vi "MultiTool-Track-Generate-ndipolarisFileOutput-Q-vectors-Accepts Joystick Command with Time Display-Testing time diff with tick.vi"() -> ()   [LabVIEW 2013]
panel:
  out "TIME":string
  out "bytes written":i32
  out "Return time string":string
  out "Length":u8
  out "Command":u8
  out "Tool 2":T1={"Port Handle"="", "Frame Number"=0, "Tx"=0.0, "Ty"=0.0, "Tz"=0.0, "Q0"=0.0, "Qx"=0.0, "Qy"=0.0, "Qz"=0.0, "Deviation"=0.0, " Markers Missing"=TRUE, "Out of Volume"=TRUE} {"Deviation" format="%#.4f"; "Qz" format="%#.4f"; "Qy" format="%#.4f"; "Qx" format="%#.4f"; "Q0" format="%#.4f"; "Tz" format="%#.2f"; "Ty" format="%#.2f"; "Tx" format="%#.2f"}
  in  "Location of ROM File for Tool 2":path=path "C:/Program Files (x86)/Northern Digital Inc/8700339.rom"
  in  "NDI  Running":bool=TRUE
  out "Stop Reading":bool=TRUE
  out "Start Reading":bool
  out "Object Identifier":string="0"
  in  "Track Outside Measurement Volume? (F:No)":bool
  in  "Track Stray Markers? (F:No)":bool
  out "Tool 1":T1={"Port Handle"="", "Frame Number"=0, "Tx"=0.0, "Ty"=0.0, "Tz"=0.0, "Q0"=0.0, "Qx"=0.0, "Qy"=0.0, "Qz"=0.0, "Deviation"=0.0, " Markers Missing"=TRUE, "Out of Volume"=TRUE} {"Deviation" format="%#.4f"; "Qz" format="%#.4f"; "Qy" format="%#.4f"; "Qx" format="%#.4f"; "Q0" format="%#.4f"; "Tz" format="%#.2f"; "Ty" format="%#.2f"; "Tx" format="%#.2f"}
  out "TCP loop":i32
  in  "TCP Server Running":bool=TRUE
  in  "Output Directory":path=path "C:/Users/Diogo/Desktop/NDI-Labview Gripper"
  out "NDI Loop":i32
  in  "VISA resource name":refnum<visa-resource-name>="COM8"
  in  "Reset? (T:Yes)":bool=TRUE
  in  "Location of ROM File for Tool 1":path=path "C:/Program Files (x86)/Northern Digital Inc/8700449.rom"
  in  "Serial Configuration":T2={"Baud Rate (9600)"=9600, "Flow Control (0:None)"=0, "Parity"=0, "Data Bits"=8, "Stop Bits"=10} {"Stop Bits" items=["1.0"=10, "2.0"=20]; "Parity" items=["None", "Odd", "Even"]; "Flow Control (0:None)" items=["None", "XON/XOFF"]; "Baud Rate (9600)" items=["9600"=9600, "14.4k"=14400, "19.2k"=19200, "38.4k"=38400, "57.6k "=57600, "115.2k"=115200]}
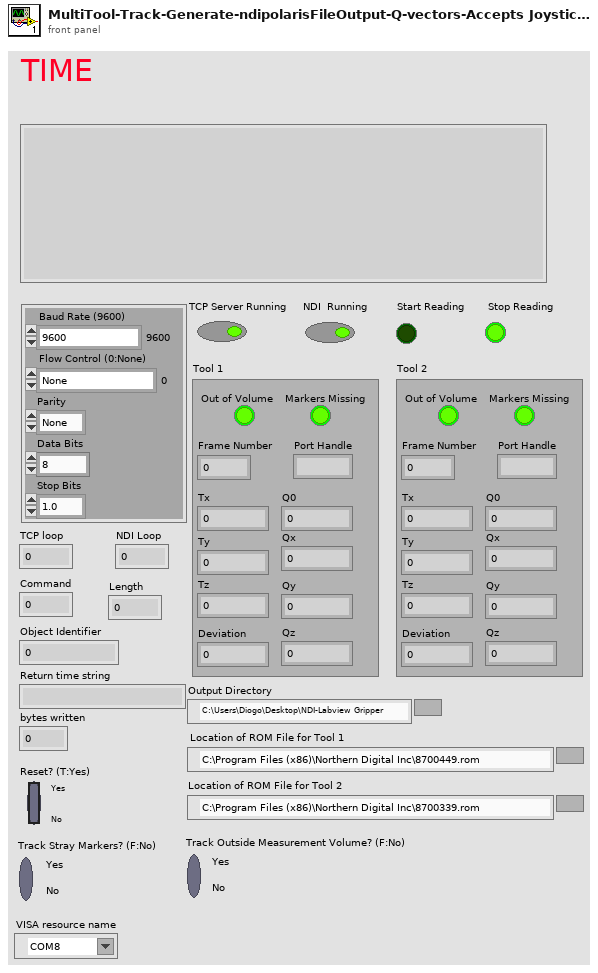
[diagram p1: front panel]
types:
  T1 = cluster{"Port Handle":string, "Frame Number":i32, "Tx":dbl, "Ty":dbl, "Tz":dbl, "Q0":dbl, "Qx":dbl, "Qy":dbl, "Qz":dbl, "Deviation":dbl, " Markers Missing":bool, "Out of Volume":bool}
  T2 = cluster{"Baud Rate (9600)":u32, "Flow Control (0:None)":u16, "Parity":u16, "Data Bits":u16, "Stop Bits":u16}
  T3 = cluster{"Port Handle":string, "Frame Number":u32, "Tx":dbl, "Ty":dbl, "Tz":dbl, "Q0":dbl, "Qx":dbl, "Qy":dbl, "Qz":dbl, "Deviation":dbl, "Missing?":bool, "Out of Volume?":bool}[]
  T4 = cluster{"Transformations[0]":cluster{"Port Handle":string, "Frame Number":u32, "Tx":dbl, "Ty":dbl, "Tz":dbl, "Q0":dbl, "Qx":dbl, "Qy":dbl, "Qz":dbl, "Deviation":dbl, "Missing?":bool, "Out of Volume?":bool}, "Transformations[1]":cluster{"Port Handle":string, "Frame Number":u32, "Tx":dbl, "Ty":dbl, "Tz":dbl, "Q0":dbl, "Qx":dbl, "Qy":dbl, "Qz":dbl, "Deviation":dbl, "Missing?":bool, "Out of Volume?":bool}, "Transformations[2]":cluster{"Port Handle":string, "Frame Number":u32, "Tx":dbl, "Ty":dbl, "Tz":dbl, "Q0":dbl, "Qx":dbl, "Qy":dbl, "Qz":dbl, "Deviation":dbl, "Missing?":bool, "Out of Volume?":bool}, "Transformations[3]":cluster{"Port Handle":string, "Frame Number":u32, "Tx":dbl, "Ty":dbl, "Tz":dbl, "Q0":dbl, "Qx":dbl, "Qy":dbl, "Qz":dbl, "Deviation":dbl, "Missing?":bool, "Out of Volume?":bool}, "Transformations[4]":cluster{"Port Handle":string, "Frame Number":u32, "Tx":dbl, "Ty":dbl, "Tz":dbl, "Q0":dbl, "Qx":dbl, "Qy":dbl, "Qz":dbl, "Deviation":dbl, "Missing?":bool, "Out of Volume?":bool}, "Transformations[5]":cluster{"Port Handle":string, "Frame Number":u32, "Tx":dbl, "Ty":dbl, "Tz":dbl, "Q0":dbl, "Qx":dbl, "Qy":dbl, "Qz":dbl, "Deviation":dbl, "Missing?":bool, "Out of Volume?":bool}, "Transformations[6]":cluster{"Port Handle":string, "Frame Number":u32, "Tx":dbl, "Ty":dbl, "Tz":dbl, "Q0":dbl, "Qx":dbl, "Qy":dbl, "Qz":dbl, "Deviation":dbl, "Missing?":bool, "Out of Volume?":bool}, "Transformations[7]":cluster{"Port Handle":string, "Frame Number":u32, "Tx":dbl, "Ty":dbl, "Tz":dbl, "Q0":dbl, "Qx":dbl, "Qy":dbl, "Qz":dbl, "Deviation":dbl, "Missing?":bool, "Out of Volume?":bool}, "Transformations[8]":cluster{"Port Handle":string, "Frame Number":u32, "Tx":dbl, "Ty":dbl, "Tz":dbl, "Q0":dbl, "Qx":dbl, "Qy":dbl, "Qz":dbl, "Deviation":dbl, "Missing?":bool, "Out of Volume?":bool}}
  T5 = cluster{"Port Handle":string, "Frame Number":u32, "Tx":dbl, "Ty":dbl, "Tz":dbl, "Q0":dbl, "Qx":dbl, "Qy":dbl, "Qz":dbl, "Deviation":dbl, "Missing?":bool, "Out of Volume?":bool}
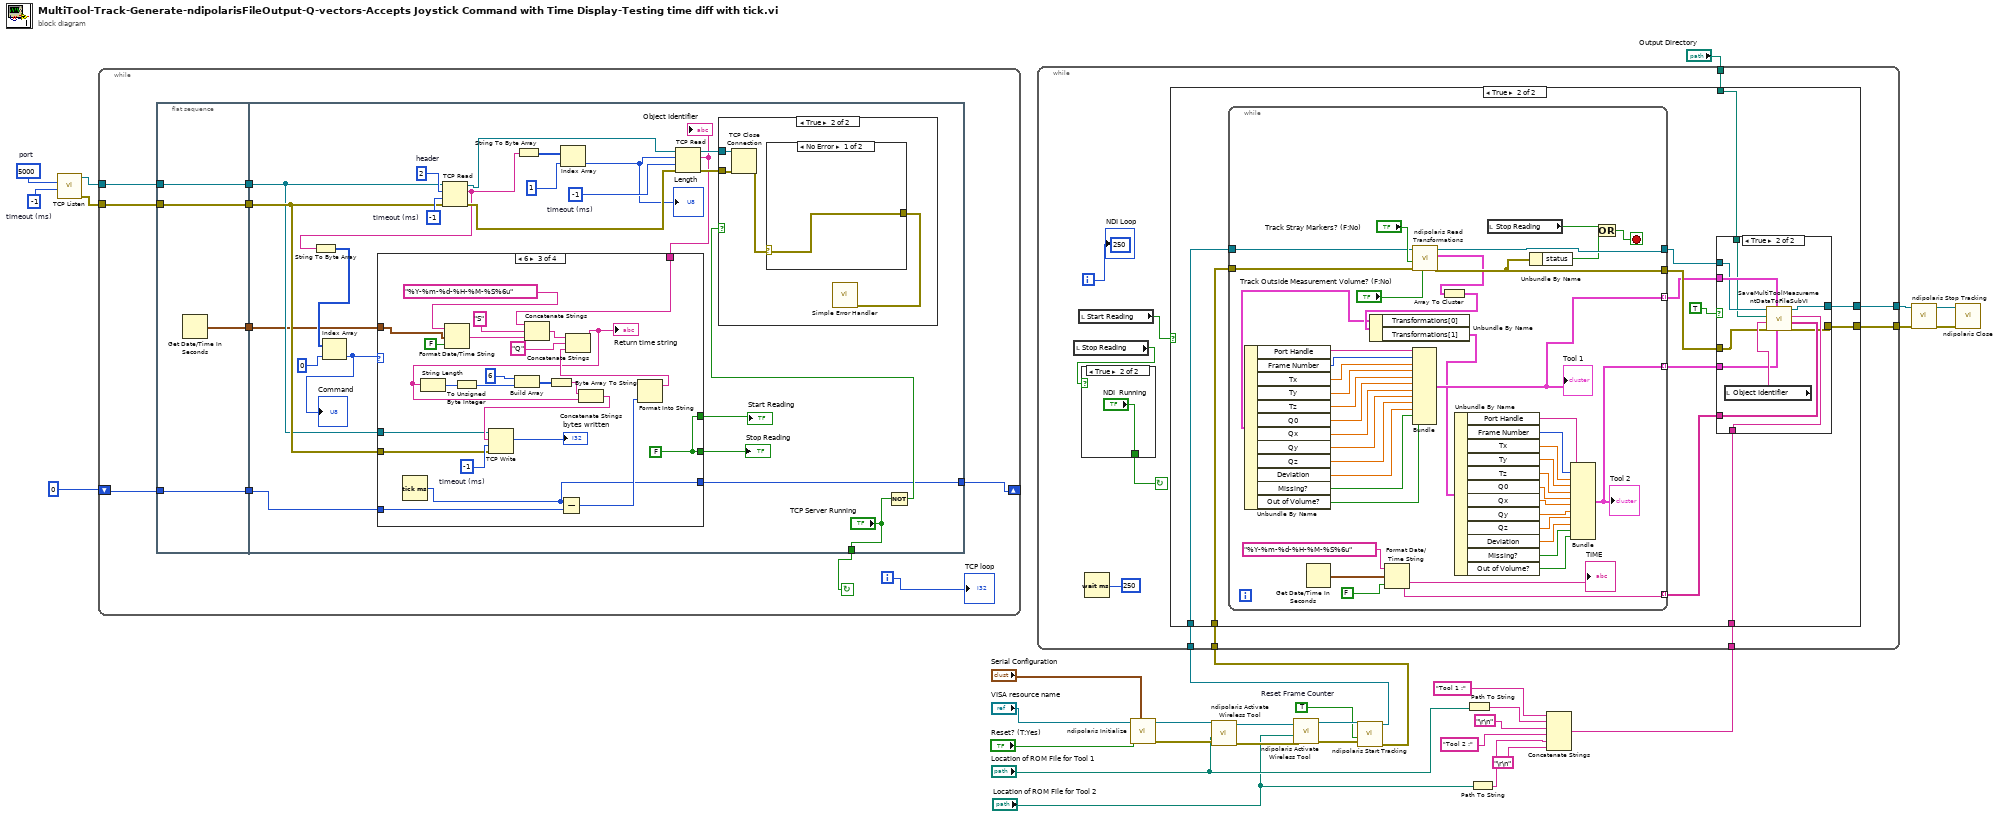
[diagram p0: block diagram]
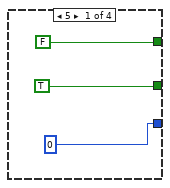
[diagram p2: hidden frame]
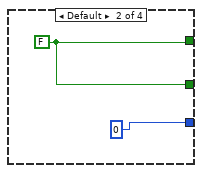
[diagram p3: hidden frame]
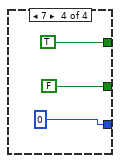
[diagram p4: hidden frame]
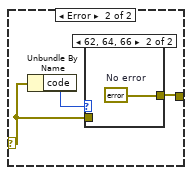
[diagram p6: hidden frame]
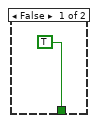
[diagram p8: hidden frame]
diagram:
  w22 = TRUE  # Reset Frame Counter
  w31 = u16 5000  # port
  w30 = i8 -1  # timeout (ms)
  n1 = call <vilib>:"TCP Listen.vi"("timeout ms (wait forever: -1)"=w30, "port"=w31) -> ("error out"=w25:errorcluster, "connection ID"=w26:refnum<k5>)  [unwired: 5 in, 3 out]
  n2 = while {
    tunnel: w26 -> [w39]
    tunnel: w25 -> [w40]
    shift-right: [w32] -> _
    shift-left: u32 0 -> [w34]
    i -> [w35]
    stop <- w41 continue-if-true
    n3 = flat-sequence {
      tunnel: w39 -> [w44]
      tunnel: w40 -> [w45]
      tunnel: [w45] -> w38
      tunnel: [w44] -> w37
      tunnel: [w43] -> w36
      tunnel: w34 -> [w42]
      tunnel: [w42] -> w33
      tunnel: ["TCP Server Running"] -> w41
      tunnel: w38 -> [w51]
      tunnel: w37 -> [w49]
      tunnel: w36 -> [w48]
      tunnel: w33 -> [w47]
      tunnel: [w46] -> w32
      frame #0 {
        n4 = Get Date/Time In Seconds() -> (seconds since 1Jan1904=w43:timestamp)
      }
      frame #1 {
        w65 = i8 -1  # timeout (ms)
        w68 = i8 -1  # timeout (ms)
        w69 = i8 2  # header
        n5 = TCP Read(connection ID=w49, bytes to read=w69, error in (no error)=w51, 9:w68) -> (connection ID out=w67:refnum<k5>, data out=w56:string, error out=w66:errorcluster)  [unwired: 1 in]
        n6 = String To Byte Array(string=w56) -> (unsigned byte array=w59:u8[])
        n7 = Index Array(array=w59, index=0) -> (element=w52:u8)
        "Command" <- w52
        n8 = String To Byte Array(string=w56) -> (unsigned byte array=w58:u8[])
        n9 = Index Array(array=w58, index=1) -> (element=w55:u8)
        "Length" <- w55
        n10 = TCP Read(connection ID=w67, bytes to read=w55, error in (no error)=w66, 9:w65) -> (connection ID out=w64:refnum<k5>, data out=w50:string, error out=w63:errorcluster)  [unwired: 1 in]
        "Object Identifier" <- w50
        n11 = case shown="6" w52 {
          tunnel: [FALSE w74 w84 TRUE] -> w62
          tunnel: [TRUE w74 w84 FALSE] -> w61
          tunnel: w51 -> [_ _ w87 _]
          tunnel: w50 -> [_ _ w86 _]
          tunnel: w49 -> [_ _ w85 _]
          tunnel: w48 -> [_ _ w83 _]
          tunnel: w47 -> [_ _ w76 _]
          tunnel: [u32 0 u32 0 w75 u32 0] -> w46
          frame 5 {
          }
          frame Default {
            w74 = FALSE
          }
          frame 6 {
            w95 = i8 -1  # timeout (ms)
            w84 = FALSE
            n12 = Tick Count (ms)() -> (millisecond timer value=w75:u32)
            n13 = Format Date/Time String(time format string (%c)="%Y-%m-%d-%H-%M-%S%6u", seconds (now)=w83, UTC format=FALSE) -> (date/time string=w98:string)
            n14 = Concatenate Strings(w86, "S", w98) -> (w82:string)
            n15 = Subtract(x=w75, y=w76) -> (x-y=w77:u32)
            n16 = Format Into String(w77) -> (resulting string=w80:string)  [unwired: 3 in, 1 out]
            n17 = Concatenate Strings(w82, "Q", w80) -> (w79:string)
            "Return time string" <- w79
            n18 = String Length(string=w79) -> (length=w92:i32)
            n19 = To Unsigned Byte Integer(number=w92) -> (unsigned 8bit integer=w91:u8)
            n20 = Build Array(u8 6, w91) -> (w89:u8[])
            n21 = Byte Array To String(unsigned byte array=w89) -> (string=w94:string)
            n22 = Concatenate Strings(w94, w79) -> (w88:string)
            n23 = TCP Write(connection ID=w85, data in=w88, error in (no error)=w87, 9:w95) -> (bytes written=→"bytes written":i32)  [unwired: 2 out]
          }
          frame 7 {
          }
        }
        "Start Reading" <- w62
        "Stop Reading" <- w61
        n24 = Not(x="TCP Server Running") -> (.not. x?=w53:bool)
        n25 = case shown="True" w53 {
          tunnel: w64 -> [_ w103]
          tunnel: w63 -> [_ w102]
          frame False {
          }
          frame True {
            n26 = TCP Close Connection(connection ID=w103, error in (no error)=w102) -> (error out=w104:errorcluster)  [unwired: 1 in, 1 out]
            n27 = case shown="No Error" w104 {
              selector: w104 -> [w106 w108]
              tunnel: [w106 w107] -> w105
              frame No Error {
              }
              frame Error {
                n28 = Unbundle By Name(w108) -> ("code"=w109:i32)
                n29 = case shown="62, 64, 66" w109 {
                  tunnel: w108 -> [w110 _]
                  tunnel: [w110 w111] -> w107
                  frame Default {
                  }
                  frame 62, 64, 66 {
                    w111 = errorcluster {"status"=FALSE, "code"=0, "source"=""}  # No error
                  }
                }
              }
            }
            n30 = call <vilib>:"Simple Error Handler.vi"("error in (no error)"=w105) -> ()  [unwired: 1 in, 8 out]
          }
        }
      }
    }
    "TCP loop" <- w35
  }
  n31 = call <instrlib>:"ndipolaris Initialize.vi"("Serial Configuration"="Serial Configuration", "Reset? (T: Yes)"="Reset? (T:Yes)", "VISA resource name"="VISA resource name") -> ("error out"=w12:errorcluster, "VISA resource name out"=w13:refnum<visa-resource-name>)  [unwired: 7 in]
  n32 = call <instrlib>:"ndipolaris Activate Wireless Tool.vi"("error in (no error)"=w12, "Location of ROM File for Tool"="Location of ROM File for Tool 1", "VISA resource name"=w13) -> ("error out"=w10:errorcluster, "VISA resource out"=w11:refnum<visa-resource-name>)  [unwired: 6 in, 1 out]
  n33 = call <instrlib>:"ndipolaris Activate Wireless Tool.vi"("error in (no error)"=w10, "Location of ROM File for Tool"="Location of ROM File for Tool 2", "VISA resource name"=w11) -> ("error out"=w23:errorcluster, "VISA resource out"=w24:refnum<visa-resource-name>)  [unwired: 6 in, 1 out]
  n34 = call <instrlib>:"ndipolaris Start Tracking.vi"("error in (no error)"=w23, "Reset Frame Counter? (F:No)"=w22, "VISA resource name"=w24) -> ("error out"=w17:errorcluster, "VISA resource out"=w21:refnum<visa-resource-name>)  [unwired: 7 in]
  n35 = Path To String(path="Location of ROM File for Tool 1") -> (string=w6:string)
  n36 = Path To String(path="Location of ROM File for Tool 2") -> (string=w4:string)
  n37 = Concatenate Strings("Tool 1 :" ("string"), w6, "\r\n", "Tool 2 :" ("string"), w4, "\r\n") -> (w14:string)
  n38 = while {
    tunnel: w21 -> [w121]
    tunnel: [w120] -> w18
    tunnel: w17 -> [w119]
    tunnel: "Output Directory" -> [w118]
    tunnel: [w117] -> w15
    tunnel: w14 -> [w113]
    i -> [w122]
    stop <- w112 continue-if-true
    (unwired) u8 250
    n39 = local read "Stop Reading"() -> (w114:bool)
    n40 = local read "Start Reading"() -> (w115:bool)
    n41 = case shown="True" w114 {
      tunnel: [TRUE "NDI  Running"] -> w112
      frame False {
      }
      frame True {
      }
    }
    n42 = Wait (ms)(milliseconds to wait=u32 250) -> ()  [unwired: 1 out]
    n43 = case shown="True" w115 {
      tunnel: w121 -> [w126 w138]
      tunnel: [w126 w134] -> w120
      tunnel: w119 -> [w125 w137]
      tunnel: w118 -> [_ w136]
      tunnel: [w125 w133] -> w117
      tunnel: w113 -> [_ w128]
      frame False {
      }
      frame True {
        n44 = while {
          tunnel: [w192] -> w130
          tunnel: [w191] -> w135
          tunnel: [w168] -> w131 mode=indexing
          tunnel: [w169] -> w132 mode=indexing
          tunnel: w138 -> [w167]
          tunnel: w137 -> [w166]
          tunnel: [w151] -> w127 mode=indexing
          stop <- w193 stop-if-true
          n45 = Get Date/Time In Seconds() -> (seconds since 1Jan1904=w172:timestamp)
          n46 = Format Date/Time String(time format string (%c)="%Y-%m-%d-%H-%M-%S%6u", seconds (now)=w172, UTC format=FALSE) -> (date/time string=w169:string)
          "TIME" <- w169
          n47 = call <instrlib>:"ndipolaris Read Transformations.vi"("Track Outside Measurement Volume? (F:No)"="Track Outside Measurement Volume? (F:No)", "error in (no error)"=w166, "Track Stray Markers? (F:No)"="Track Stray Markers? (F:No)", "VISA resource name"=w167) -> ("error out"=w191:errorcluster, "Transformations"=w176:T3, "VISA resource out"=w192:refnum<visa-resource-name>)  [unwired: 4 in, 1 out]
          n48 = Array To Cluster(array=w176) -> (cluster=w187:T4)
          n49 = Unbundle By Name(w187) -> ("Transformations[0]"=w186:T5, "Transformations[1]"=w164:T5)
          n50 = Unbundle By Name(w186) -> ("Port Handle"=w185:string, "Frame Number"=w184:u32, "Tx"=w183:dbl, "Ty"=w182:dbl, "Tz"=w181:dbl, "Q0"=w180:dbl, "Qx"=w179:dbl, "Qy"=w178:dbl, "Qz"=w177:dbl, "Deviation"=w175:dbl, "Missing?"=w174:bool, "Out of Volume?"=w173:bool)
          n51 = Bundle("Port Handle"=w185, "Frame Number"=w184, "Tx"=w183, "Ty"=w182, "Tz"=w181, "Q0"=w180, "Qx"=w179, "Qy"=w178, "Qz"=w177, "Deviation"=w175, "Missing?"=w174, "Out of Volume?"=w173) -> (w168:T5)  [unwired: 1 in]
          "Tool 1" <- w168
          n52 = Unbundle By Name(w164) -> ("Port Handle"=w163:string, "Frame Number"=w162:u32, "Tx"=w161:dbl, "Ty"=w160:dbl, "Tz"=w159:dbl, "Q0"=w158:dbl, "Qx"=w157:dbl, "Qy"=w156:dbl, "Qz"=w155:dbl, "Deviation"=w154:dbl, "Missing?"=w153:bool, "Out of Volume?"=w152:bool)
          n53 = local read "Stop Reading"() -> (w165:bool)
          n54 = Unbundle By Name(w191) -> ("status"=w190:bool)
          n55 = Bundle("Port Handle"=w163, "Frame Number"=w162, "Tx"=w161, "Ty"=w160, "Tz"=w159, "Q0"=w158, "Qx"=w157, "Qy"=w156, "Qz"=w155, "Deviation"=w154, "Missing?"=w153, "Out of Volume?"=w152) -> (w151:T5)  [unwired: 1 in]
          "Tool 2" <- w151
          n56 = Or(x=w165, y=w190) -> (x .or. y?=w193:bool)
        }
        n57 = case shown="True" TRUE {
          tunnel: w136 -> [_ w148]
          tunnel: w135 -> [w139 w146]
          tunnel: [w140 w145] -> w134
          tunnel: [w139 w141] -> w133
          tunnel: w132 -> [_ w144]
          tunnel: w131 -> [_ w150]
          tunnel: w130 -> [w140 w149]
          tunnel: w128 -> [_ w143]
          tunnel: w127 -> [_ w142]
          frame False {
          }
          frame True {
            n58 = local read "Object Identifier"() -> (w147:string)
            n59 = call "SaveMultiToolMeasurementDataToFileSubVI.vi"("Array of Time for Measurement"=w144, "NDI Tool"=w143, "Array - Transformations of Tool 2"=w142, "Array - Transformations of Tool 1"=w150, "error in (no error)"=w146, "Object number"=w147, "Output Directory"=w148, "VISA Refnum in"=w149) -> ("error out"=w141:errorcluster, "VISA Refnum out"=w145:refnum<visa-resource-name>)
          }
        }
      }
    }
    "NDI Loop" <- w122
  }
  n60 = call <instrlib>:"ndipolaris Stop Tracking.vi"("error in (no error)"=w15, "VISA resource name"=w18) -> ("error out"=w19:errorcluster, "VISA resource out"=w20:refnum<visa-resource-name>)  [unwired: 8 in]
  n61 = call <instrlib>:"ndipolaris Close.vi"("error in (no error)"=w19, "VISA resource name"=w20) -> ()  [unwired: 9 in, 1 out]
